vi "Start.vi"(8 "error in (no error)":errorcluster, 10 "Container":refnum<vi>, 11 "ArrayManager in":refnum<class "ArrayManager.lvclass">) -> (0 "error out":errorcluster, 3 "ArrayManager out":refnum<class "ArrayManager.lvclass">)   [LabVIEW 2020, in "OOPanel.lvlib" / "ArrayManager.lvclass"]
uses:
  ArrayManager.lvclass
  Array Panel Async.vi
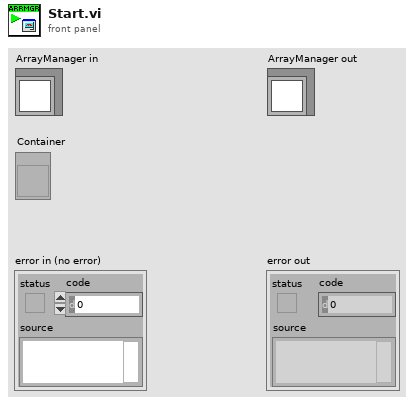
[diagram p1: front panel]
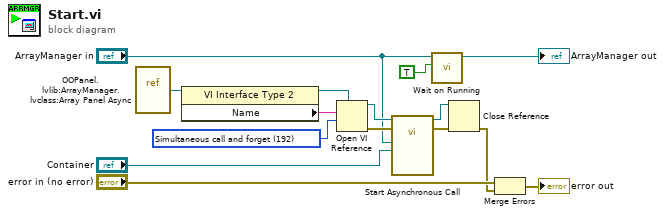
[diagram p0: block diagram]
diagram:
  w9 = 192 items=["Record modifications"=1, "Open templates for editing"=2, "Prompt user to save"=4, "Prepare for reentrant run"=8, "Prompt to find missing subVIs"=16, "Hide loading dialog box"=32, "Enable simultaneous calls"=64, "Prepare to call and forget"=128, "Simultaneous call and forget"=192, "Prepare to call and collect"=256, "Simultaneous call and collect"=320]
  n1 = vi-ref "OOPanel.lvlib:ArrayManager.lvclass:Array Panel Async.vi"() -> (w7:refnum<vi>)
  n2 = property class="VI Interface Type 2"(reference=w7) -> (reference out=w10:refnum<vi>, "Name"=w8:string)  [unwired: 1 in, 1 out]
  n3 = Open VI Reference(type specifier VI Refnum (for type only)=w10, vi path=w8, options=w9) -> (vi reference=w12:refnum<vi>, error out=w11:errorcluster)  [unwired: 3 in]
  n4 = call-by-ref "Start Asynchronous Call"(reference=w12, error in=w11, "Container"="Container", "PanelArray in"="ArrayManager in") -> (reference out=w14:refnum<vi>, error out=w13:errorcluster)  [unwired: 10 in]
  n5 = call "Wait on Running.vi"("Value"=TRUE, "ArrayManager in"="ArrayManager in") -> ("ArrayManager out"=→"ArrayManager out":refnum<class "ArrayManager.lvclass">)  [unwired: 8 in, 1 out]
  n6 = Close Reference(reference=w14, error in (no error)=w13) -> (error out=w1:errorcluster)
  n7 = Merge Errors("error in (no error)", w1) -> (→"error out":errorcluster)
